vi "Read Mass.vi"(8 "error in (no error)":errorcluster, 11 "PhysicsComponent in":refnum<class "PhysicsComponent.lvclass">) -> (0 "error out":errorcluster, 2 "Mass out":sgl, 3 "PhysicsComponent out":refnum<class "PhysicsComponent.lvclass">)   [LabVIEW 2022 SP3, in "PhysicsComponent.lvclass"]
uses:
  PhysicsComponent.lvclass
  PhysicsComponent.lvclass/PhysicsComponent.ctl
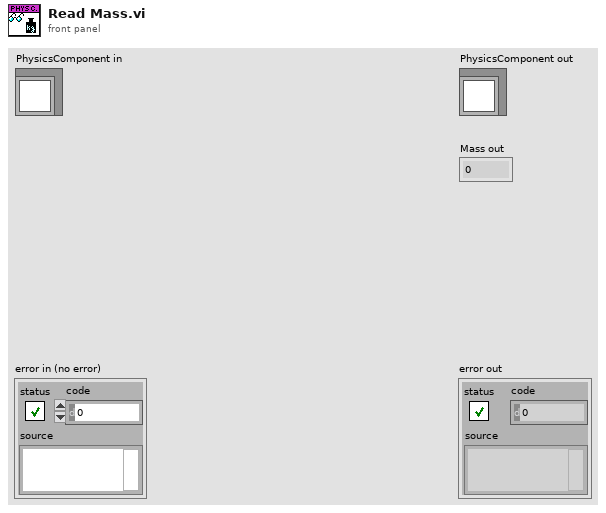
[diagram p1: front panel]
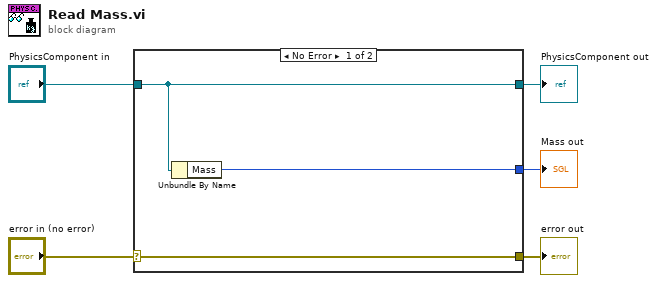
[diagram p0: block diagram]
diagram:
  n1 = case shown="No Error" "error in (no error)" {
    selector: "error in (no error)" -> [w8 w9]
    tunnel: [w8 w9] -> w4
    tunnel: [w7 w10] -> w2
    tunnel: "PhysicsComponent in" -> [w7 w10]
    tunnel: [w6 _] -> w1
    frame No Error {
      n2 = Unbundle By Name(w7) -> ("Mass"=w6:i16)
    }
    frame Error {
    }
  }
  "error out" <- w4
  "PhysicsComponent out" <- w2
  "Mass out" <- w1
